vi "ACT_LabVIEW1_Task3B_Team072.vi"() -> ()   [LabVIEW 2016]
uses:
  <vilib>/express/express arith-compare/Formula/XNode/ExpressFormulaBlockNode.xnode
panel:
  out "a":dbl
  in  "T (F)":dbl
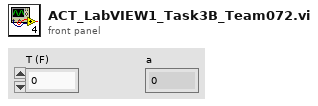
[diagram p1: front panel]
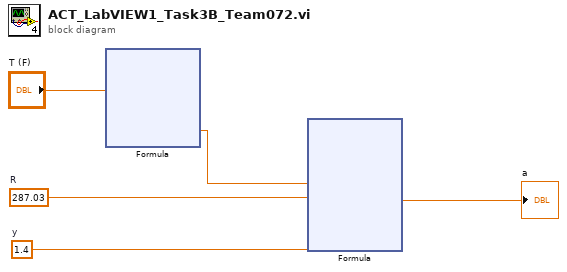
[diagram p0: block diagram]
diagram:
  w2 = 1.4  # y
  w3 = 287.03  # R
  n1 = xnode "Formula"("T"="T (F)") -> ("Result"=w4:dbl)  [unwired: 1 in, 1 out]
  n2 = xnode "Formula"("T"=w4, "R"=w3, "y"=w2) -> ("Result"=→"a":dbl)  [unwired: 1 in, 1 out]
